vi "Find Example Parents Directory.vi"(8 "error in (no error)":errorcluster) -> (0 "error out":errorcluster, 1 "Exists":bool, 2 "TestStand Format Furnace Control Example Root Dir":string, 3 "Furnace Control Example Root Directory":path, 5 "TestStand Examples Relative Path":string)   [LabVIEW 2015]
doc: "Find the parent directory for the example. TestStand needs this information to properly call VIs in the application.\n____\nDelacor QMH Thermal Chamber Examples 4.0.0.21\nCopyright (c) 2018, Delacor"
uses:
  <vilib>/Utility/error.llb/Error Cluster From Error Code.vi
  <vilib>/ErrorRing/Error Ring.xnode
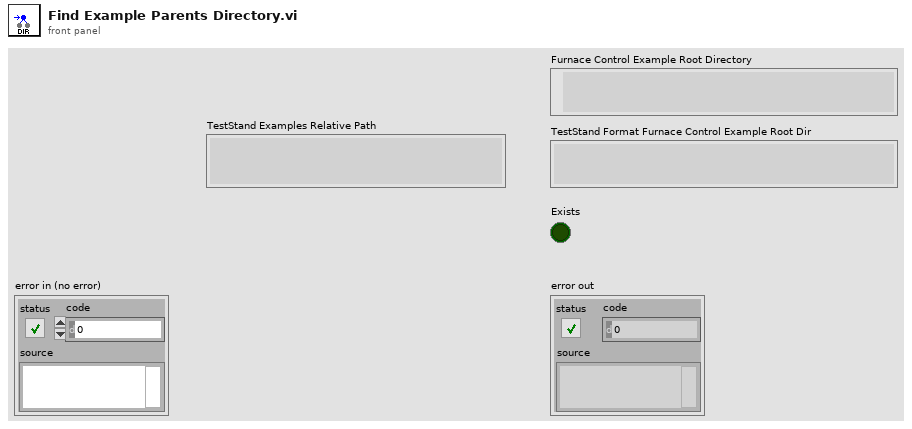
[diagram p1: front panel]
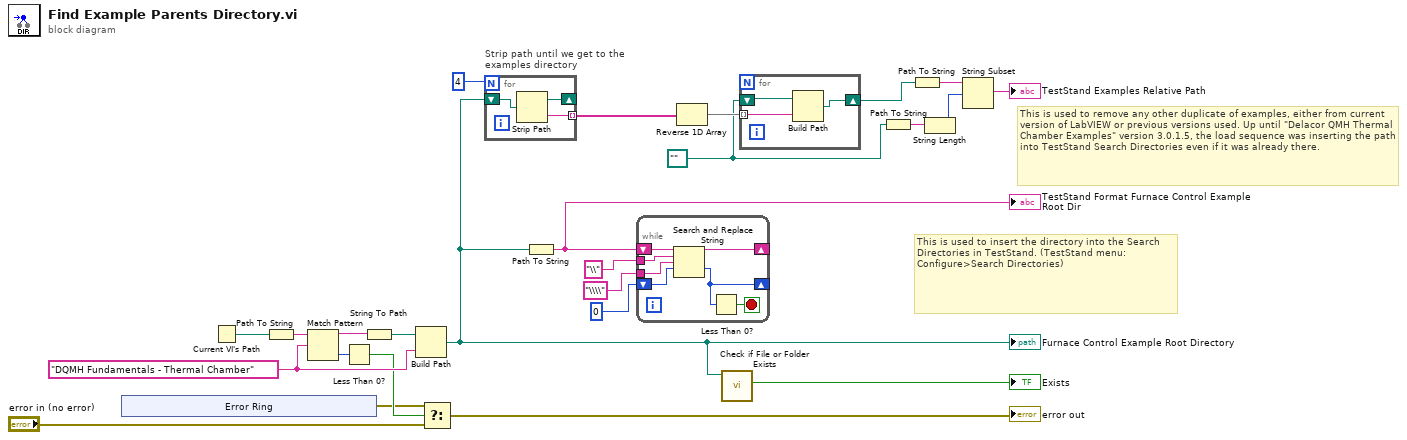
[diagram p0: block diagram]
diagram:
  w4 = path ".." ("appended path")
  w21 = "DQMH Fundamentals - Thermal Chamber"
  # "This is used to remove any other duplicate of examples, either from current version of LabVIEW or previous versions used. Up until \"Delacor QMH Thermal Chamber Examples\" version 3.0.1.5, the load sequence was inserting the path into TestStand Search Directories even if it was already there."
  # "This is used to insert the directory into the Search Directories in TestStand. (TestStand menu: Configure>Search Directories)"
  n1 = xnode "Error Ring"() -> ("error out"=w18:errorcluster)
  n2 = Current VI's Path() -> (path=w25:path)
  n3 = Path To String(path=w25) -> (string=w24:string)
  n4 = Match Pattern(string=w24, regular expression=w21) -> (before substring=w23:string, offset past match=w20:i32)  [unwired: 1 in, 2 out]
  n5 = Less Than 0?(x=w20) -> (x < 0?=w19:bool)
  n6 = String To Path(string=w23) -> (path=w22:path)
  n7 = Build Path(base path=w22, name or relative path=w21) -> (appended path=w10:path)
  "Furnace Control Example Root Directory" <- w10
  n8 = Select(t=w18, s=w19, f="error in (no error)") -> (s? t:f=→"error out":errorcluster)
  n9 = for "Strip path until we get to the \nexamples directory" {
    N: 4 -> [_]
    shift-right: [w27] -> _
    shift-left: w10 -> [w28]
    tunnel: [w26] -> w7 mode=indexing
    n10 = Strip Path(path=w28) -> (stripped path=w27:path, name=w26:string)
  }
  n11 = Path To String(path=w10) -> (string=w11:string)
  "TestStand Format Furnace Control Example Root Dir" <- w11
  n12 = while {
    tunnel: "\\" -> [w34]
    tunnel: "\\\\" -> [w33]
    shift-right: [w32] -> _
    shift-left: w11 -> [w35]
    shift-right: [w29] -> _
    shift-left: 0 -> [w31]
    stop <- w30 stop-if-true
    n13 = Search and Replace String(input string=w35, search string=w34, replace string=w33, offset=w31) -> (result string=w32:string, offset past replacement=w29:i32)  [unwired: 4 in, 2 out]
    n14 = Less Than 0?(x=w29) -> (x < 0?=w30:bool)
  }
  n15 = Reverse 1D Array(array=w7) -> (reversed array=w6:string[])
  n16 = call <vilib>:"Check if File or Folder Exists.vi"("path"=w10) -> ("file or folder exists?"=→"Exists":bool)  [unwired: 8 in, 2 out]
  n17 = for {
    tunnel: w6 -> [w37] mode=indexing
    shift-right: [w36] -> w5
    shift-left: w4 -> [w38]
    n18 = Build Path(base path=w38, name or relative path=w37) -> (appended path=w36:path)
  }
  n19 = Path To String(path=w4) -> (string=w3:string)
  n20 = Path To String(path=w5) -> (string=w8:string)
  n21 = String Length(string=w3) -> (length=w1:i32)
  n22 = String Subset(string=w8, offset (0)=w1) -> (substring=→"TestStand Examples Relative Path":string)  [unwired: 1 in]
